vi "GenerateAPIEvent_GIS Printer.vi"(6 "Timeout (ms)":u32=600000, 7 "Wait (F)":bool, 8 "error in (no error)":errorcluster, 9 "Task ID":string, 10 "API Command Cluster":T1, 11 "GIS Printer in":refnum<class "GIS Printer.lvclass">) -> (0 "error out":errorcluster, 1 "Aborted":bool, 2 "TimedOut":bool, 3 "GIS Printer out":refnum<class "GIS Printer.lvclass">)   [LabVIEW 2022 SP3, in "GIS Printer.lvclass"]
uses:
  GIS Printer.lvclass
  Typedefs/API Command Cluster.ctl
  Typedefs/API Command Enum.ctl
  Typedefs/API Event Data.ctl
  Typedefs/API Task State.ctl
  <vilib>/event_ctls.llb/usereventprio.ctl
  GIS Printer.lvclass/GIS Printer.ctl
panel:
  out "Return Value":variant
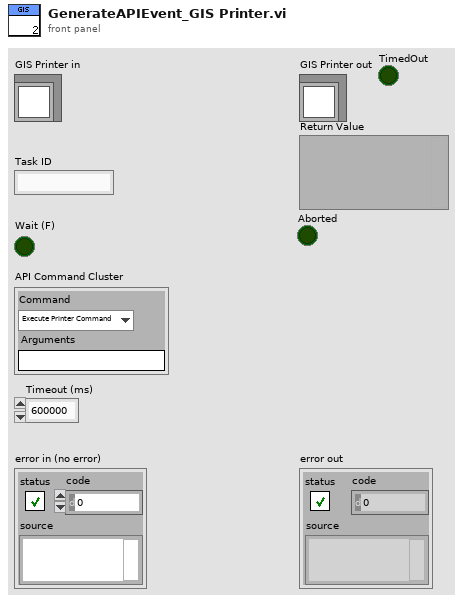
[diagram p1: front panel]
types:
  T1 = typedef "GIS Printer.lvclass/API Command Cluster.ctl" = cluster{"Command":T2, "Arguments":string}
  T2 = typedef "GIS Printer.lvclass/API Command Enum.ctl" = enum16{"Execute Printer Command", "Abort"}
  T3 = typedef "usereventprio.ctl" = enum32{"high priority", "normal priority"}
  T4 = typedef "GIS Printer.lvclass/API Task State.ctl" = enum16{"Completed", "Errored", "Pending"}
  T5 = typedef "GIS Printer.lvclass/API Event Data.ctl" = cluster{"Task":cluster{"Time Stamp":timestamp, "Timeout (ms)":u32, "Task State":T4, "Task Error":errorcluster, "Task ID":string}, "Command":variant, "Return Value":variant}
  T6 = typedef "GIS Printer.lvclass/Private Data.ctl" = cluster{"UserEvents":T7, "All Dependencies":cluster{"Class References":refnum<class>[], "Class Names":string[]}, "PrinterConiguration":T8, "Status":T9, "GISHeadStatus":T10[], "HeadStatus":T11}
  T7 = typedef "GIS Printer.lvclass/UserEvents.ctl" = cluster{"API Incoming Event":refnum<user-event>, "API Executed Event":refnum<user-event>, "API Return Event":refnum<user-event>, "Status Changed Event":refnum<user-event>, "Abort":refnum<user-event>, "stop process":refnum<user-event>, "GISPollStatus":refnum<user-event>, "GISHeadStatus":refnum<user-event>}
  T8 = typedef "GIS Printer.lvclass/PrinterConfiguration--Cluster.ctl" = cluster{"IPAddress":string, "Move Stage on RTP Command?":bool, "Stage Move Position":string, "PH1-Prime Path":path, "PH2-Prime Path":path, "PH3-Prime Path":path, "PH4-Prime Path":path, "PH5-Prime Path":path, "PH6-Prime Path":path, "PrintScriptsFolder":path, "PurgeScriptsFolder":path, "StageScriptsFolder":path, "PH1-HeatOn Path":path, "PH2-HeatOn Path":path, "PH3-HeatOn Path":path, "PH4-HeatOn Path":path, "PH5-HeatOn Path":path, "PH6-HeatOn Path":path, "PH1-HeatOff Path":path, "PH2-HeatOff Path":path, "PH3-HeatOff Path":path, "PH4-HeatOff Path":path, "PH5-HeatOff Path":path, "PH6-HeatOff Path":path}
  T9 = typedef "GIS Printer.lvclass/Status Cluster.ctl" = cluster{"Command Status":variant, "TCP Commands & Responses":string[][], "Printer Busy?":bool}
  T10 = typedef "GIS Status--Cluster.ctl" = cluster{"HeadEnabled":bool, "SpitEnabled":bool, "HeaterEnabled":bool, "TargetTemperature":dbl, "CurrentTemperature":dbl}
  T11 = typedef "HeadEnableStatus--cluster.ctl" = cluster{"PH1_Enable":bool, "PH2_Enable":bool, "PH3_Enable":bool, "PH4_Enable":bool, "PH5_Enable":bool, "PH6_Enable":bool}
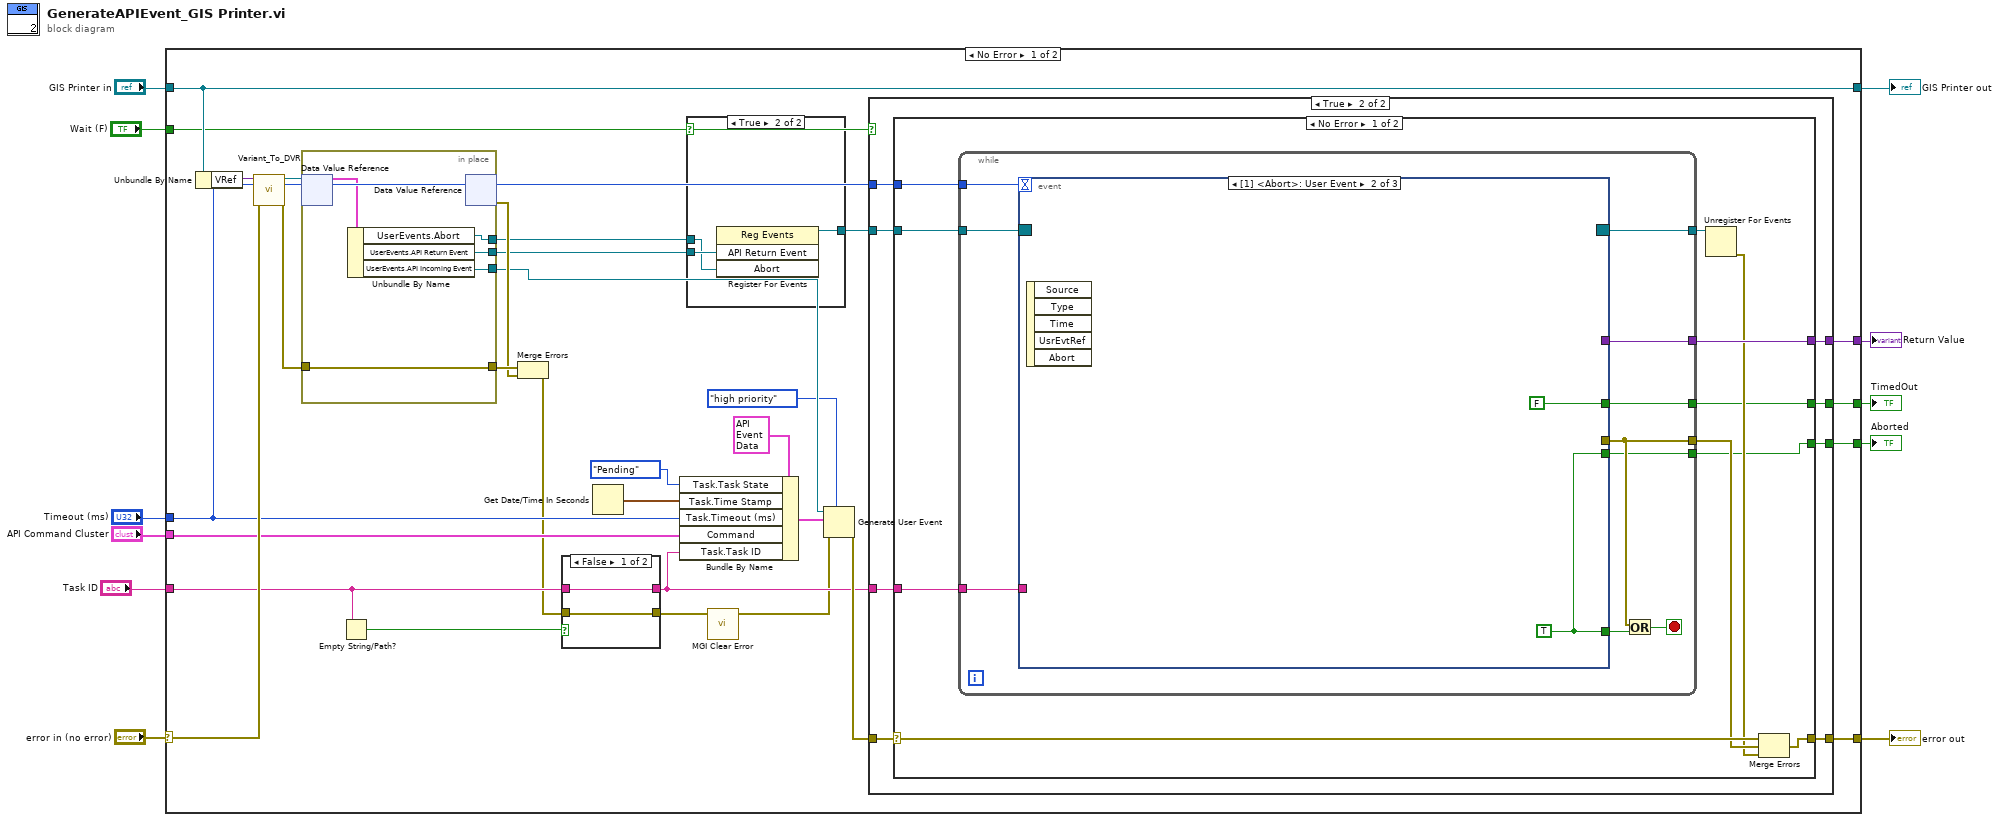
[diagram p0: block diagram]
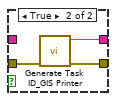
[diagram p2: hidden frame]
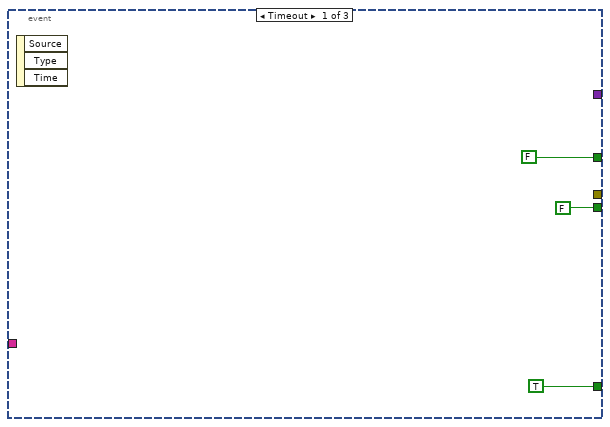
[diagram p4: hidden frame]
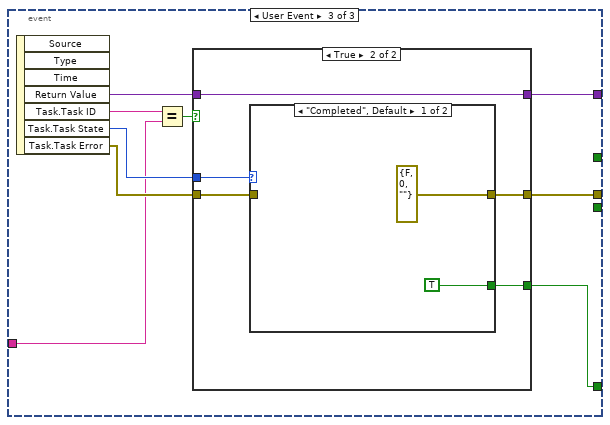
[diagram p5: hidden frame]
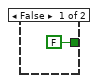
[diagram p6: hidden frame]
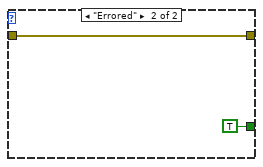
[diagram p7: hidden frame]
diagram:
  n1 = case shown="No Error" "error in (no error)" {
    selector: "error in (no error)" -> [w41 w111]
    tunnel: [w22 w111] -> w10
    tunnel: [w35 w110] -> w8
    tunnel: "GIS Printer in" -> [w35 w110]
    tunnel: "Wait (F)" -> [w28 _]
    tunnel: "Timeout (ms)" -> [w26 _]
    tunnel: "API Command Cluster" -> [w29 _]
    tunnel: [w23 _] -> w4
    tunnel: "Task ID" -> [w20 _]
    tunnel: [w16 _] -> w2
    tunnel: [w12 _] -> w1
    frame No Error {
      n2 = Unbundle By Name(w35) -> ("VRef"=w40:variant)
      n3 = call "Variant_To_DVR.vi"("error in (no error)"=w41, "Variant"=w40) -> ("error out"=w38:errorcluster, "DVR"=w39:refnum<data-value>)  [unwired: 8 in]
      n4 = in-place {
        in-place-border: w38 -> [w108]
        in-place-border: [w108] -> w37
        in-place-border: [w107] -> w34
        in-place-border: [w106] -> w33
        in-place-border: [w105] -> w13
        n5 = in-place-dvr #1(w39) -> (w109:T6)  [unwired: 1 out]
        n6 = Unbundle By Name(w109) -> ("UserEvents.Abort"=w105:refnum<user-event>, "UserEvents.API Return Event"=w107:refnum<user-event>, "UserEvents.API Incoming Event"=w106:refnum<user-event>)
        n7 = in-place-dvr #1() -> (w36:errorcluster)  [unwired: 1 in, 1 out]
      }
      n8 = Empty String/Path?(string/path=w20) -> (empty?=w21:bool)
      n9 = Merge Errors(w37, w36) -> (w19:errorcluster)
      n10 = case shown="False" w21 {
        tunnel: [w43 w46] -> w17
        tunnel: w20 -> [w43 _]
        tunnel: w19 -> [w42 w45]
        tunnel: [w42 w44] -> w18
        frame False {
        }
        frame True {
          n11 = call "Generate Task ID_GIS Printer.vi"("error in (no error)"=w45) -> ("error out"=w44:errorcluster, "Task ID"=w46:string)  [unwired: 9 in]
        }
      }
      n12 = Get Date/Time In Seconds() -> (seconds since 1Jan1904=w31:timestamp)
      n13 = Bundle By Name(cluster=T5 {"Task"={"Time Stamp"=timestamp(0 s since 1904-01-01), "Timeout (ms)"=0, "Task State"=enum."Completed", "Task Error"={"status"=FALSE, "code"=0, "source"=""}, "Task ID"=""}, "Command"=variant, "Return Value"=variant} ("event data"), "Task.Task State"=API_Task_State."Pending", "Task.Time Stamp"=w31, "Task.Timeout (ms)"=w26, "Command"=w29, "Task.Task ID"=w17) -> (w30:T5)
      n14 = case shown="True" w28 {
        tunnel: w34 -> [_ w104]
        tunnel: [_ w103] -> w25
        tunnel: w13 -> [_ w102]
        frame False {
        }
        frame True {
          n15 = register-events(w104, w102) -> (reference out=w103:refnum<event-registration>)  [unwired: 2 in, 1 out]
        }
      }
      n16 = call <userlib>:"MGI Clear Error.vi"("Error In"=w18) -> ("Error Out"=w15:errorcluster)  [unwired: 6 in]
      n17 = Generate User Event(priority (normal)=usereventprio."high priority", user event=w33, event data cluster=w30, error in=w15) -> (error out=w27:errorcluster)  [unwired: 1 out]
      n18 = case shown="True" w28 {
        tunnel: w27 -> [w47 w55]
        tunnel: w26 -> [_ w54]
        tunnel: w25 -> [_ w53]
        tunnel: [_ w52] -> w23
        tunnel: [w47 w51] -> w22
        tunnel: w17 -> [_ w50]
        tunnel: [_ w49] -> w16
        tunnel: [_ w48] -> w12
        frame False {
        }
        frame True {
          n19 = case shown="No Error" w55 {
            selector: w55 -> [w62 w101]
            tunnel: w54 -> [w66 _]
            tunnel: w53 -> [w65 _]
            tunnel: [w64 _] -> w52
            tunnel: [w59 w101] -> w51
            tunnel: w50 -> [w58 _]
            tunnel: [w57 _] -> w49
            tunnel: [w56 _] -> w48
            frame No Error {
              n20 = while {
                tunnel: w66 -> [w76]
                tunnel: w65 -> [w75]
                tunnel: [w74] -> w64
                tunnel: [w71] -> w63
                tunnel: [w70] -> w61
                tunnel: w58 -> [w69]
                tunnel: [w68] -> w57
                tunnel: [w67] -> w56
                stop <- w72 stop-if-true
                n21 = event shown="[1] <Abort>: User Event" {
                  selector: w75 -> [_ _ _]
                  dyn-events: [_ _ _] -> w71
                  timeout: w76 -> [_ _ _]
                  tunnel: [_ _ w85] -> w74
                  tunnel: [_ _ w84] -> w70
                  tunnel: [TRUE w80 w82] -> w73
                  tunnel: w69 -> [_ _ w83]
                  tunnel: [FALSE FALSE _] -> w68
                  tunnel: [FALSE w80 _] -> w67
                  event Timeout {
                    n22 = event-data() -> ()  [unwired: 1 in, 3 out]
                  }
                  event User Event {
                    w80 = TRUE
                    n23 = event-data() -> ()  [unwired: 1 in, 5 out]
                  }
                  event User Event {
                    n24 = event-data() -> ("Return Value"=w86:variant, "Task.Task ID"=w90:string, "Task.Task State"=w88:T4, "Task.Task Error"=w87:errorcluster)  [unwired: 1 in, 3 out]
                    n25 = Equal?(x=w90, y=w83) -> (x = y?=w89:bool)
                    n26 = case shown="True" w89 {
                      tunnel: w88 -> [_ w96]
                      tunnel: w87 -> [_ w95]
                      tunnel: [_ w94] -> w85
                      tunnel: w86 -> [_ w94]
                      tunnel: [_ w93] -> w84
                      tunnel: [FALSE w92] -> w82
                      frame False {
                      }
                      frame True {
                        n27 = case shown="\"Completed\", Default" w96 {
                          tunnel: w95 -> [_ w100]
                          tunnel: [errorcluster {"status"=FALSE, "code"=0, "source"=""} ("Task Error") w100] -> w93
                          tunnel: [TRUE TRUE] -> w92
                          frame "Completed", Default {
                          }
                          frame "Errored" {
                          }
                        }
                      }
                    }
                  }
                }
                n28 = Or(x=w70, y=w73) -> (x .or. y?=w72:bool)
              }
              n29 = Unregister For Events(event registration refnum=w63) -> (error out=w60:errorcluster)  [unwired: 1 in]
              n30 = Merge Errors(w62, w61, w60) -> (w59:errorcluster)
            }
            frame Error {
            }
          }
        }
      }
    }
    frame Error {
    }
  }
  "error out" <- w10
  "GIS Printer out" <- w8
  "Return Value" <- w4
  "TimedOut" <- w2
  "Aborted" <- w1
